vi "IT6322_Variable.vi"(9 "TestIndex":u8, 10 "IT6322_Port_List":refnum<visa-resource-name>[](array[refnum]), 11 "模式":enum16{"Write", "Read"}(ring)) -> (1 "IT6322_COM":refnum<visa-resource-name>)   [LabVIEW 2015, in "IT6322.lvlib"]
uses:
  IT6322.lvlib
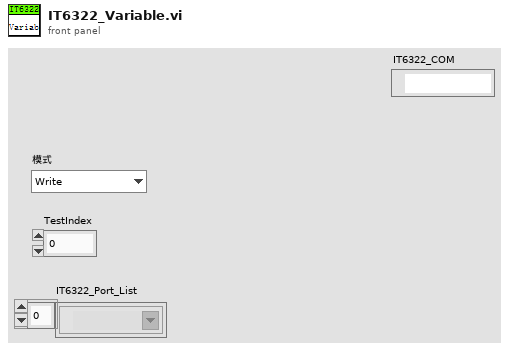
[diagram p1: front panel]
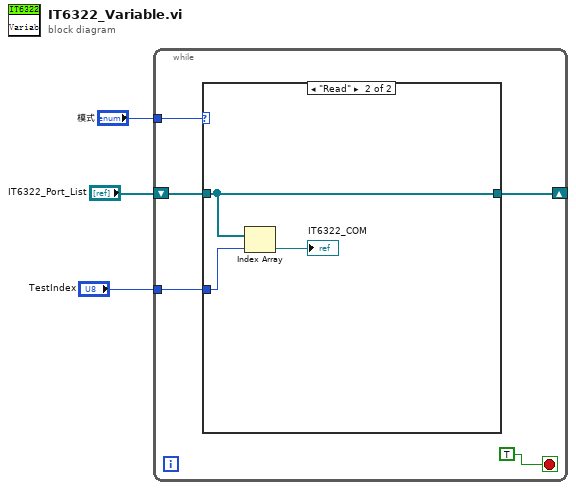
[diagram p0: block diagram]
diagram:
  n1 = while {
    tunnel: "模式" -> [w8]
    shift-right: [w5] -> _
    shift-left: "IT6322_Port_List" -> [w7]
    tunnel: "TestIndex" -> [w4]
    stop <- TRUE stop-if-true
    n2 = case shown="\"Read\"" w8 {
      tunnel: w7 -> [w9 w12]
      tunnel: [w9 w12] -> w5
      tunnel: w4 -> [_ w11]
      frame "Write", Default {
      }
      frame "Read" {
        n3 = Index Array(array=w12, index=w11) -> (element=→"IT6322_COM":refnum<visa-resource-name>)
      }
    }
  }
